vi "Main.vi"() -> ()   [LabVIEW 2019, in "MainController.lvlib"]
doc: "This Continuous Measurement sample project is based on the Queued Message Handler template.\n\nThe Event Handling Loop generates messages based on user interface actions.\n\nThe Message Handling Loop processes messages generated by the Event Handling Loop, or by other messages. There are also Acquisition and Logging message handling loop subVIs, and a chart updating loop."
uses:
  MainController/MainController.lvlib
  MainController/Cluster - MainData.ctl
  MainController/All Message Queues.ctl
  MainController/Cluster - MainControllerMessage.ctl
  MainController/Enum - MainState.ctl
  AutoMode/Cluster - AutoModeMessage.ctl
  AutoMode/Enum - AutoModeState.ctl
  ManualMode/Cluster - ManualModeMessageCluster.ctl
  ManualMode/Enum - ManualModeMessage.ctl
  Settings/CTL_MessageCluster.ctl
  Settings/CTL_SettingsMessage.ctl
  MainController/Cluster - HardwareConfiguration.ctl
  MainController/Cluster - LoggingConfiguration.ctl
  MainController/Cluster - TestSettings.ctl
  MainController/UI State.ctl
  MainController/UI Data.ctl
  Settings/Cluster - Settings.ctl
  <vilib>/Utility/error.llb/DialogType.ctl
  <vilib>/Utility/error.llb/Error Cluster From Error Code.vi
  <vilib>/ErrorRing/Error Ring.xnode
  Settings/Settings.lvlib
  support/User Event - Stop/User Event - Stop.lvlib
  ManualMode/ManualMode.lvlib
  AutoMode/AutoMode.lvlib
  support/User Interface/UserInterface.lvlib
  Dialogs/Flyout/Flyout.lvlib
panel:
  in  "ManualMode":bool
  in  "Test Report":bool
  in  "AutoMode":bool
  in  "HiliteNav":bool
  out "NavPaneTitle":string
  in  "Back":bool
  in  "Exit":bool
  in  "Global Navigation":bool
  in  "Settings":bool
  in  "COM":refnum<visa-resource-name>
  out "Mark 10":bool
  in  "Connect":bool
  in  "Titlebar":bool
  in  "Maximize":bool
  in  "Minimize":bool
  in  "Close":bool
  in  "CommandBar":T1
  out "Auto Mode":bool
  # "Auto Mode"
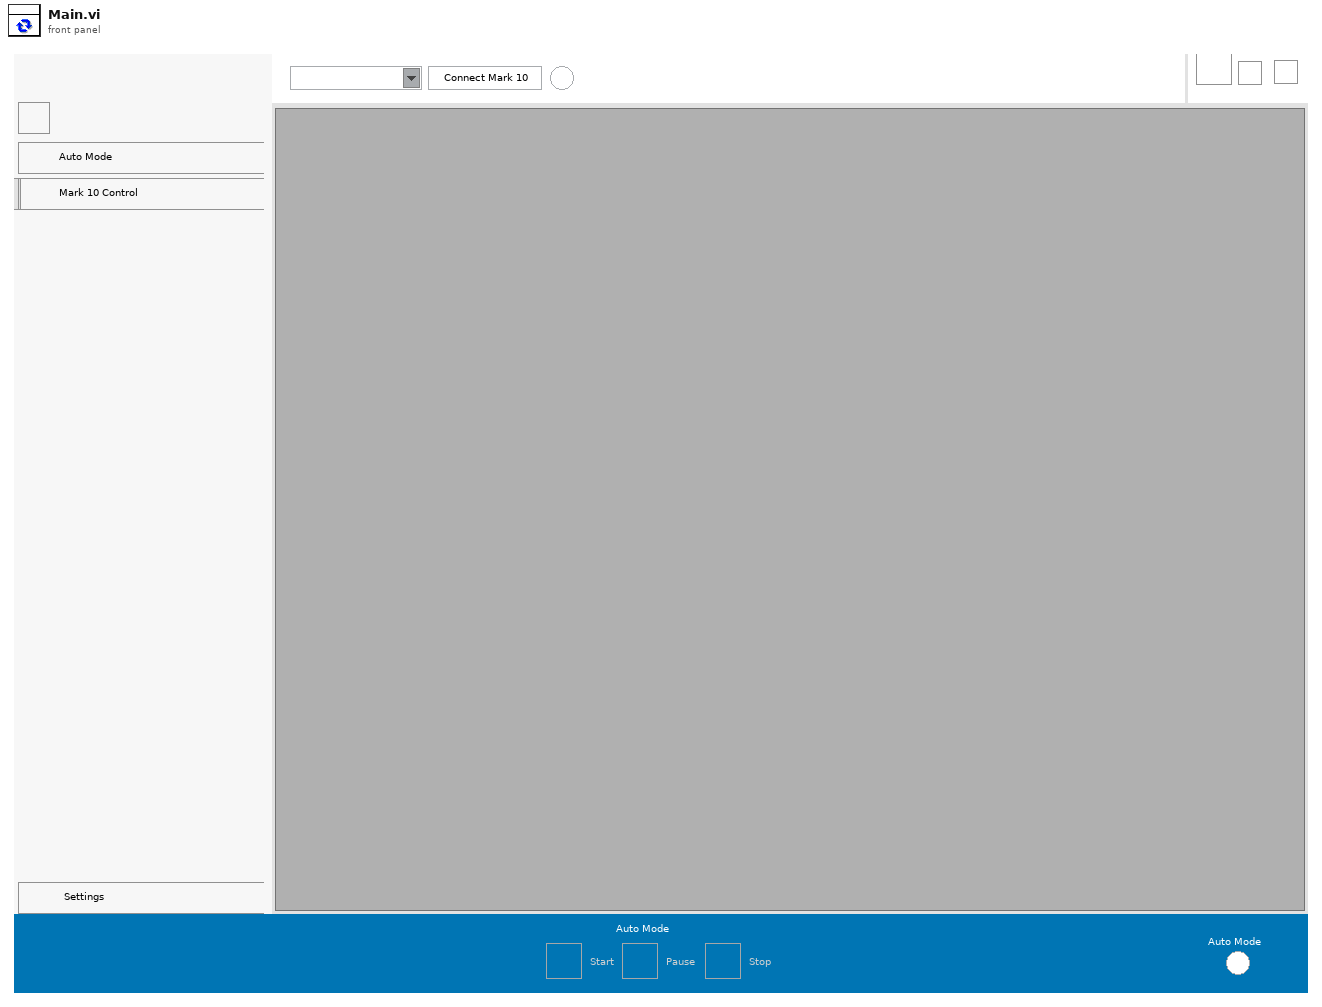
[diagram p1: front panel]
types:
  T1 = cluster{"StartCycleTest":bool, "PauseCycleTest":bool, "StopCycleTest":bool}
  T2 = typedef "MainController.lvlib/Cluster - MainData.ctl" = cluster{"MessageQueues":T3, "HardwareConfig":T4, "LoggingConfig":T5, "TestSettings":T6, "UI State":T7, "UIRefs":T8}
  T3 = typedef "MainController.lvlib/All Message Queues.ctl" = cluster{"Main":refnum<queue>, "AutoMode":refnum<queue>, "ManualMode":refnum<queue>, "Settings":refnum<queue>}
  T4 = typedef "MainController.lvlib/Cluster - HardwareConfiguration.ctl" = cluster{"Mark10COM":refnum<visa-resource-name>, "IsConnected":bool}
  T5 = typedef "MainController.lvlib/Cluster - LoggingConfiguration.ctl" = cluster{"Log File Base Path":path, "Comments ":string, "Operator":string, "File Name":string, "Description":string}
  T6 = typedef "MainController.lvlib/Cluster - TestSettings.ctl" = cluster{"Sample":u32, "Applicator Prefix":string, "Winding Distance":dbl, "Winding Speed":dbl, "Dwell Time":dbl, "Auto Increment Sample":bool, "Output Data Path":path, "File Base Path":path, "Manual Return To Zero":bool}
  T7 = typedef "MainController.lvlib/UI State.ctl" = enum16{"Idle", "AutoIdle", "AutoRunning", "ManualMode", "Settings"}
  T8 = typedef "MainController.lvlib/UI Data.ctl" = cluster{"Start Ref":refnum<vi>, "Stop Ref":refnum<vi>, "Settings Ref":refnum<vi>, "Subpanel":refnum<vi>, "HiliteNav Ref":refnum<vi>, "PauseCycle":refnum<vi>, "Connect":refnum<vi>, "ConnectionFbk":refnum<vi>, "AutoMode":refnum<vi>, "ManualMode":refnum<vi>}
  T9 = typedef "MainController.lvlib/Enum - MainState.ctl" = enum16{"Initialize", "InitUIRefs", "LaunchSettings", "LaunchAutoMode", "LaunchManualMode", "LaunchTestReport", "ConnectHardware", "DisconnectHardware", "HiliteNavItems", "StartAutoMode", "PauseAutoMode", "StopAutoMode", "ShowFlyout", "HideFlyout", "BroadcastSettings", "PickupTestSettings", "BroadcastHW", "AutoTestDone", "DAQStatus", "UpdateCommandBar", "Error", "RecieveError", "Exit"}
  T10 = enum32{"Invalid", "Standard", "Closed", "Hidden", "Minimized", "Maximized"}
  T11 = typedef "AutoMode.lvlib/Enum - AutoModeState.ctl" = enum16{"Initialize", "Idle", "UpdateConfig", "UpdateHWConfig", "BroadcastSettings", "Start", "CheckValidReportPath", "Winding", "WaitForWinding", "Unwind", "WaitForUnwind", "Stop", "Abort", "WriteDataToFile", "EventTriggered", "GenerateFilePath", "ZeroPosition", "GotoZero", "Error", "Exit"}
  T12 = typedef "Settings.lvlib/Cluster - Settings.ctl" = cluster{"Hardware Configuration":T4, "TestSettings":T6}
  T13 = typedef "ManualMode.lvlib/Enum - ManualModeMessage.ctl" = enum16{"Initialize", "Idle", "Start", "Stop", "Pause", "Resume", "BroadcastPreCollection", "MoveCCW", "MoveCW", "StopMove", "SetZero", "GotoZero", "UpdateHW", "SendMark10Cmd", "ReadPosition", "ReadTorque", "ReadStatus", "Error", "Exit"}
  T14 = typedef "Settings.lvlib/CTL_SettingsMessage.ctl" = enum16{"Inititalize", "Idle", "LoadSettings", "SaveSettings", "Exit"}
  T15 = typedef "DialogType.ctl" = u16
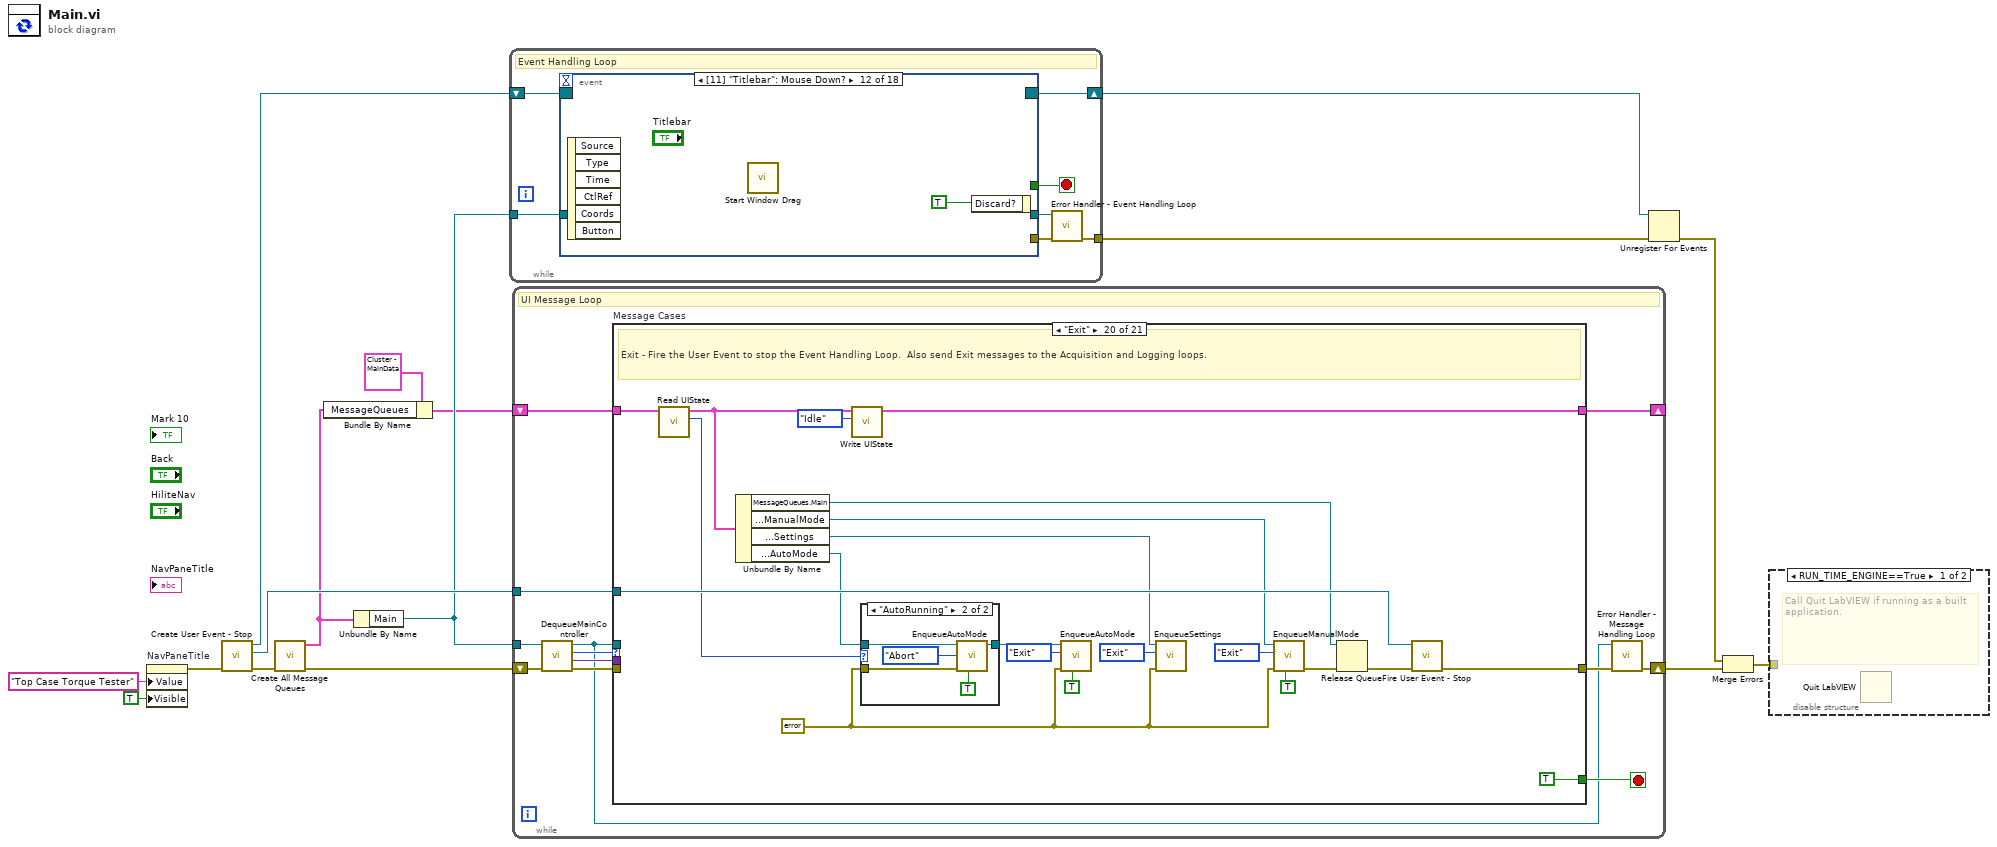
[diagram p0: block diagram]
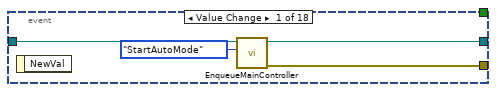
[diagram p3: hidden frame]
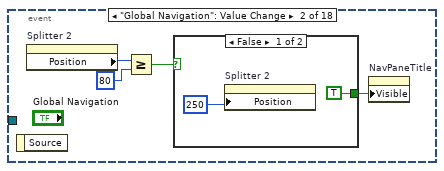
[diagram p4: hidden frame]
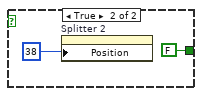
[diagram p5: hidden frame]
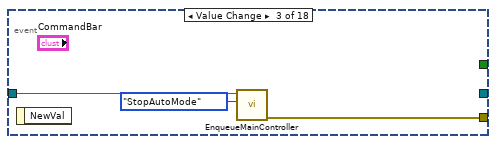
[diagram p6: hidden frame]
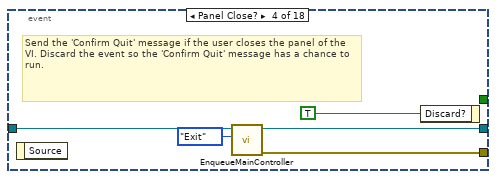
[diagram p7: hidden frame]
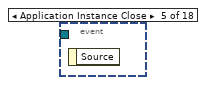
[diagram p8: hidden frame]
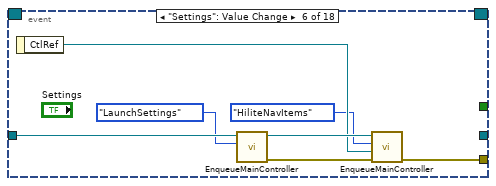
[diagram p9: hidden frame]
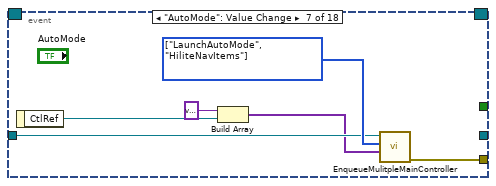
[diagram p10: hidden frame]
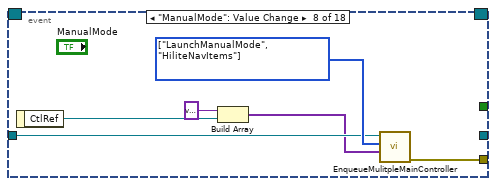
[diagram p11: hidden frame]
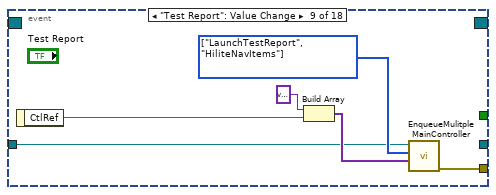
[diagram p12: hidden frame]
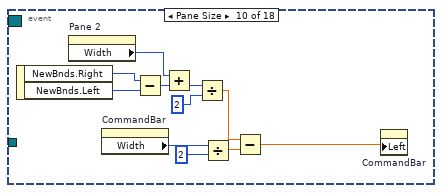
[diagram p13: hidden frame]
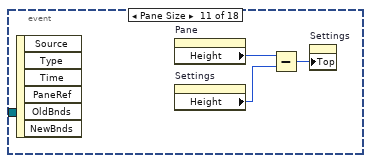
[diagram p14: hidden frame]
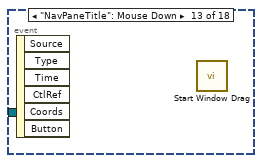
[diagram p15: hidden frame]
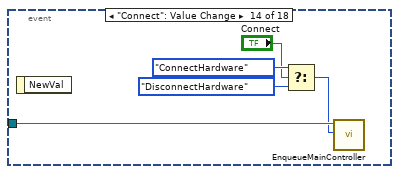
[diagram p16: hidden frame]
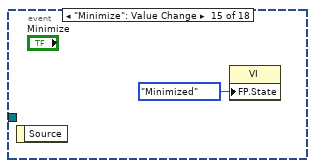
[diagram p17: hidden frame]
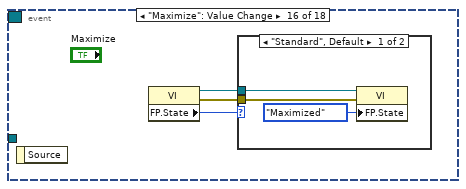
[diagram p18: hidden frame]
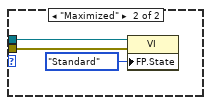
[diagram p19: hidden frame]
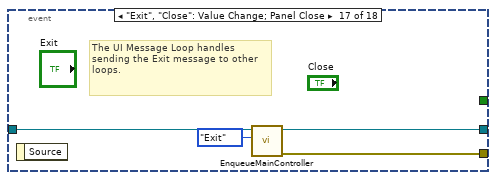
[diagram p20: hidden frame]
diagram:
  n1 = property on="NavPaneTitle" class="Str"("Value"="Top Case Torque Tester" ("NavPaneTitle"), "Visible"=TRUE) -> (error out=w5:errorcluster)  [unwired: 2 in, 1 out]
  n2 = call "Create User Event - Stop.vi"("error in (no error)"=w5) -> ("error out"=w12:errorcluster, "User Event - Stop"=w13:refnum<user-event>, "Stop Event Registration Refnum"=w14:refnum<event-registration>)  [unwired: 8 in]
  n3 = call "Create All Message Queues.vi"("error in (no error)"=w12) -> ("error out"=w7:errorcluster, "Message Queues out"=w3:T3)  [unwired: 9 in]
  n4 = Bundle By Name(cluster=T2 {"MessageQueues"={"Main"=refnum, "AutoMode"=refnum, "ManualMode"=refnum, "Settings"=refnum}, "HardwareConfig"={"Mark10COM"="", "IsConnected"=FALSE}, "LoggingConfig"={"Log File Base Path"=path "", "Comments "="", "Operator"="", "File Name"="", "Description"=""}, "TestSettings"={"Sample"=0, "Applicator Prefix"="", "Winding Distance"=0.0, "Winding Speed"=0.0, "Dwell Time"=0.0, "Auto Increment Sample"=FALSE, "Output Data Path"=path "", "File Base Path"=path "", "Manual Return To Zero"=FALSE}, "UI State"=enum."Idle", "UIRefs"={"Start Ref"=refnum, "Stop Ref"=refnum, "Settings Ref"=refnum, "Subpanel"=refnum, "HiliteNav Ref"=refnum, "PauseCycle"=refnum, "Connect"=refnum, "ConnectionFbk"=refnum, "AutoMode"=refnum, "ManualMode"=refnum}} ("MainData"), "MessageQueues"=w3) -> (w2:T2)
  n5 = Unbundle By Name(w3) -> ("Main"=w6:refnum<queue>)
  n6 = while {
    tunnel: w6 -> [w22]
    tunnel: [w18] -> w15
    shift-right: [w21] -> w10
    shift-left: w14 -> [w23]
    stop <- w20 stop-if-true
    # "Event Handling Loop"
    n7 = event shown="[11] \"Titlebar\": Mouse Down?" {
      selector: w23 -> [_ _ _ _ _ _ _ _ _ _ _ _ _ _ _ _ _ _]
      dyn-events: [_ _ _ _ _ _ _ _ _ _ _ _ _ _ _ _ _ _] -> w21
      timeout: _ -> [_ _ _ _ _ _ _ _ _ _ _ _ _ _ _ _ _ _]
      tunnel: [_ _ _ _ _ _ _ _ _ _ _ _ _ _ _ _ _ TRUE ("Discard?")] -> w20
      tunnel: w22 -> [w25 _ w37 w42 _ w50 w54 w60 w63 _ _ _ _ w88 _ _ w101 _]
      tunnel: [w27 _ w38 w41 _ w47 w56 w62 w68 _ _ _ _ _ _ _ w102 _] -> w19
      tunnel: [w26 _ _ w40 _ _ _ _ _ _ _ _ _ _ _ _ w99 _] -> w17
      event "CommandBar.StartCycleTest": Value Change {
        n8 = event-data() -> ()  [unwired: 1 in, 1 out]
        n9 = call "EnqueueMainController.vi"("Message"=Enum_-_MainState."StartAutoMode", "MainQueue"=w25) -> ("error out"=w27:errorcluster, "MainQueue out"=w26:refnum<queue>)  [unwired: 7 in, 1 out]
      }
      event "Global Navigation": Value Change {
        n10 = event-data() -> ()  [unwired: 1 in, 1 out]
        n11 = property on="Splitter 2" class="Splitter"() -> ("Position"=w29:i32)  [unwired: 2 in, 2 out]
        n12 = Greater Or Equal?(x=w29, y=80) -> (x >= y?=w30:bool)
        n13 = case shown="False" w30 {
          tunnel: [TRUE FALSE] -> w28
          frame False {
            n14 = property on="Splitter 2" class="Splitter"("Position"=250 ("Splitter Position")) -> ()  [unwired: 2 in, 2 out]
          }
          frame True {
            n15 = property on="Splitter 2" class="Splitter"("Position"=38 ("Splitter Position")) -> ()  [unwired: 2 in, 2 out]
          }
        }
        n16 = property on="NavPaneTitle" class="Str"("Visible"=w28) -> ()  [unwired: 2 in, 2 out]
      }
      event "CommandBar.StopCycleTest": Value Change {
        n17 = event-data() -> ()  [unwired: 1 in, 1 out]
        n18 = call "EnqueueMainController.vi"("Message"=Enum_-_MainState."StopAutoMode", "MainQueue"=w37) -> ("error out"=w38:errorcluster)  [unwired: 7 in, 2 out]
      }
      event Panel Close? {
        # "Send the 'Confirm Quit' message if the user closes the panel of the VI. Discard the event so the 'Confirm Quit' message has a chance to run."
        n19 = event-data() -> ()  [unwired: 1 in, 1 out]
        n20 = call "EnqueueMainController.vi"("Message"=Enum_-_MainState."Exit", "MainQueue"=w42) -> ("error out"=w41:errorcluster, "MainQueue out"=w40:refnum<queue>)  [unwired: 7 in, 1 out]
        n21 = event-data("Discard?"=TRUE) -> ()  [unwired: 1 in, 1 out]
      }
      event Application Instance Close {
        n22 = event-data() -> ()  [unwired: 1 in, 1 out]
      }
      event "Settings": Value Change {
        n23 = event-data() -> ("CtlRef"=w46:refnum<vi>)  [unwired: 1 in]
        n24 = call "EnqueueMainController.vi"("Message"=Enum_-_MainState."LaunchSettings", "MainQueue"=w50) -> ("error out"=w48:errorcluster, "MainQueue out"=w49:refnum<queue>)  [unwired: 7 in, 1 out]
        n25 = call "EnqueueMainController.vi"("error in (no error)"=w48, "Data"=w46, "Message"=Enum_-_MainState."HiliteNavItems", "MainQueue"=w49) -> ("error out"=w47:errorcluster)  [unwired: 5 in, 2 out]
      }
      event "AutoMode": Value Change {
        w55 = T9[] [enum."LaunchAutoMode", enum."HiliteNavItems"] items=["Initialize", "InitUIRefs", "LaunchSettings", "LaunchAutoMode", "LaunchManualMode", "LaunchTestReport", "ConnectHardware", "DisconnectHardware", "HiliteNavItems", "StartAutoMode", "PauseAutoMode", "StopAutoMode", "ShowFlyout", "HideFlyout", "BroadcastSettings", "PickupTestSettings", "BroadcastHW", "AutoTestDone", "DAQStatus", "UpdateCommandBar", "Error", "RecieveError", "Exit"] ("Messages")
        n26 = event-data() -> ("CtlRef"=w53:refnum<vi>)  [unwired: 1 in]
        n27 = Build Array(variant, w53) -> (w52:variant[])
        n28 = call "EnqueueMulitpleMainController.vi"("Data"=w52, "Messages"=w55, "MainQueue"=w54) -> ("error out"=w56:errorcluster)  [unwired: 6 in, 2 out]
      }
      event "ManualMode": Value Change {
        w61 = T9[] [enum."LaunchManualMode", enum."HiliteNavItems"] items=["Initialize", "InitUIRefs", "LaunchSettings", "LaunchAutoMode", "LaunchManualMode", "LaunchTestReport", "ConnectHardware", "DisconnectHardware", "HiliteNavItems", "StartAutoMode", "PauseAutoMode", "StopAutoMode", "ShowFlyout", "HideFlyout", "BroadcastSettings", "PickupTestSettings", "BroadcastHW", "AutoTestDone", "DAQStatus", "UpdateCommandBar", "Error", "RecieveError", "Exit"] ("Messages")
        n29 = event-data() -> ("CtlRef"=w59:refnum<vi>)  [unwired: 1 in]
        n30 = Build Array(variant, w59) -> (w58:variant[])
        n31 = call "EnqueueMulitpleMainController.vi"("Data"=w58, "Messages"=w61, "MainQueue"=w60) -> ("error out"=w62:errorcluster)  [unwired: 6 in, 2 out]
      }
      event "Test Report": Value Change {
        w67 = T9[] [enum."LaunchTestReport", enum."HiliteNavItems"] items=["Initialize", "InitUIRefs", "LaunchSettings", "LaunchAutoMode", "LaunchManualMode", "LaunchTestReport", "ConnectHardware", "DisconnectHardware", "HiliteNavItems", "StartAutoMode", "PauseAutoMode", "StopAutoMode", "ShowFlyout", "HideFlyout", "BroadcastSettings", "PickupTestSettings", "BroadcastHW", "AutoTestDone", "DAQStatus", "UpdateCommandBar", "Error", "RecieveError", "Exit"] ("Messages")
        n32 = event-data() -> ("CtlRef"=w66:refnum<vi>)  [unwired: 1 in]
        n33 = Build Array(variant, w66) -> (w65:variant[])
        n34 = call "EnqueueMulitpleMainController.vi"("Data"=w65, "Messages"=w67, "MainQueue"=w63) -> ("error out"=w68:errorcluster)  [unwired: 6 in, 2 out]
      }
      event Pane Size {
        n35 = event-data() -> ("NewBnds.Right"=w78:i16, "NewBnds.Left"=w79:i16)  [unwired: 1 in]
        n36 = property on="Pane 2" class="Pane"() -> ("Width"=w69:u32)  [unwired: 2 in, 2 out]
        n37 = property on="CommandBar" class="Clust (strict)"() -> ("Width"=w75:u32)  [unwired: 2 in, 2 out]
        n38 = Subtract(x=w78, y=w79) -> (x-y=w77:i16)
        n39 = Add(x=w69, y=w77) -> (x+y=w70:u32)
        n40 = Divide(x=w70, y=i16 2) -> (x/y=w73:dbl)
        n41 = Divide(x=w75, y=u32 2) -> (x/y=w72:dbl)
        n42 = Subtract(x=w73, y=w72) -> (x-y=w71:dbl)
        n43 = property on="CommandBar" class="Clust (strict)"("Left"=w71) -> ()  [unwired: 2 in, 2 out]
      }
      event Pane Size {
        n44 = event-data() -> ()  [unwired: 1 in, 6 out]
        n45 = property on="Pane" class="Pane"() -> ("Height"=w80:u32)  [unwired: 2 in, 2 out]
        n46 = property on="Settings" class="Bool"() -> ("Height"=w82:u32)  [unwired: 2 in, 2 out]
        n47 = Subtract(x=w80, y=w82) -> (x-y=w81:u32)
        n48 = property on="Settings" class="Bool"("Top"=w81) -> ()  [unwired: 2 in, 2 out]
      }
      event "Titlebar": Mouse Down? {
        n49 = event-data() -> ()  [unwired: 1 in, 6 out]
        n50 = call "Start Window Drag.vi"() -> ()  [unwired: 10 in, 2 out]
        n51 = event-data("Discard?"=TRUE) -> ()  [unwired: 1 in, 1 out]
      }
      event "NavPaneTitle": Mouse Down {
        n52 = event-data() -> ()  [unwired: 1 in, 6 out]
        n53 = call "Start Window Drag.vi"() -> ()  [unwired: 10 in, 2 out]
      }
      event "Connect": Value Change {
        n54 = event-data() -> ()  [unwired: 1 in, 1 out]
        n55 = Select(t=Enum_-_MainState."ConnectHardware" ("Message"), s="Connect", f=Enum_-_MainState."DisconnectHardware" ("Message")) -> (s? t:f=w84:T9)
        n56 = call "EnqueueMainController.vi"("Message"=w84, "MainQueue"=w88) -> ()  [unwired: 7 in, 3 out]
      }
      event "Minimize": Value Change {
        n57 = event-data() -> ()  [unwired: 1 in, 1 out]
        n58 = property class="VI"("FP.State"=T10."Minimized" ("Front Panel Window:State")) -> ()  [unwired: 2 in, 2 out]
      }
      event "Maximize": Value Change {
        n59 = event-data() -> ()  [unwired: 1 in, 1 out]
        n60 = property class="VI"() -> (reference out=w91:refnum<vi>, error out=w92:errorcluster, "FP.State"=w90:T10)  [unwired: 2 in]
        n61 = case shown="\"Standard\", Default" w90 {
          tunnel: w92 -> [w94 w97]
          tunnel: w91 -> [w93 w96]
          frame "Standard", Default {
            n62 = property class="VI"(reference=w93, error in=w94, "FP.State"=T10."Maximized" ("Front Panel Window:State")) -> ()  [unwired: 2 out]
          }
          frame "Maximized" {
            n63 = property class="VI"(reference=w96, error in=w97, "FP.State"=T10."Standard" ("Front Panel Window:State")) -> ()  [unwired: 2 out]
          }
        }
      }
      event "Exit", "Close": Value Change; Panel Close {
        # "The UI Message Loop handles sending the Exit message to other loops."
        n64 = event-data() -> ()  [unwired: 1 in, 1 out]
        n65 = call "EnqueueMainController.vi"("Message"=Enum_-_MainState."Exit", "MainQueue"=w101) -> ("error out"=w102:errorcluster, "MainQueue out"=w99:refnum<queue>)  [unwired: 7 in, 1 out]
      }
      event User Event {
        # "The Message Handling Loop processed an \"Exit\" message, which fired this event to stop the Event Handling Loop."
        n66 = event-data() -> ()  [unwired: 1 in, 1 out]
      }
    }
    n67 = call "Error Handler - Event Handling Loop.vi"("error in (no error)"=w19, "Message Queue"=w17) -> ("dup error in"=w18:errorcluster)  [unwired: 8 in, 1 out]
  }
  n68 = while {
    tunnel: w6 -> [w110]
    tunnel: w13 -> [w114]
    shift-right: [w107] -> w16
    shift-left: w7 -> [w113]
    shift-right: [w105] -> _
    shift-left: w2 -> [w109]
    stop <- w115 stop-if-true
    # "UI Message Loop"
    n69 = call "DequeueMainController.vi"("error in (no error)"=w113, "MainQueue"=w110) -> ("error out"=w112:errorcluster, "Data"=w111:variant, "Message"=w106:T9, "MainQueue out"=w104:refnum<queue>)  [unwired: 5 in, 1 out]
    n70 = case "Message Cases" shown="\"Exit\"" w106 {
      selector: w106 -> [_ _ _ _ _ _ _ _ _ _ _ _ _ _ _ _ _ _ _ _ w342]
      tunnel: w104 -> [_ _ _ _ _ _ _ _ _ _ _ _ _ _ _ _ w268 _ _ _ _]
      tunnel: w112 -> [w119 _ w149 w156 w161 w165 w169 w176 w181 w192 w197 w207 w212 w224 w232 _ w271 w280 w287 _ _]
      tunnel: [w118 _ w146 w155 w160 w162 w168 w175 w177 w193 w196 w201 w211 w218 w231 _ w269 w277 w284 w332 w343] -> w108
      tunnel: [_ _ _ _ _ _ _ _ _ _ _ _ _ _ _ _ _ _ _ TRUE _] -> w115
      tunnel: w111 -> [_ _ _ _ _ _ _ _ _ w189 _ w205 w210 w222 _ _ _ w279 w286 _ _]
      tunnel: w114 -> [_ _ _ _ _ _ _ _ _ _ _ _ _ _ _ _ _ _ _ w333 _]
      tunnel: [w116 w124 w147 w153 w158 w164 w166 w174 w179 w183 w194 w198 w208 w216 w226 w242 w266 w276 w281 w325 w341] -> w105
      tunnel: w109 -> [w117 w126 w148 w154 w159 w163 w167 w170 w180 w183 w194 w198 w208 w220 w230 w243 w270 w276 w281 w326 w341]
      frame "Initialize" {
        # "Initialize - Get configuration settings, then message the UI to initialize, and broadcast the settings to the other message loops."
        n71 = call "Initialize.vi"("Error In"=w119, "MainData"=w117) -> ("Error Out"=w118:errorcluster, "MainData out"=w116:T2)  [unwired: 8 in]
        n72 = property on="Pane" class="Pane"() -> ("Height"=w122:u32)  [unwired: 2 in, 2 out]
        n73 = property on="Settings" class="Bool"() -> ("Height"=w120:u32)  [unwired: 2 in, 2 out]
        n74 = Subtract(x=w122, y=w120) -> (x-y=w121:u32)
        n75 = property on="Settings" class="Bool"("Top"=w121) -> ()  [unwired: 2 in, 2 out]
      }
      frame "InitUIRefs" {
        # "Init UI Refs - Store control references for UI controls.  Also enable/disable controls appropriately."
        n76 = control-ref of="StartCycleTest"() -> (w132:refnum<vi>)
        n77 = control-ref of="PauseCycleTest"() -> (w135:refnum<vi>)
        n78 = control-ref of="StopCycleTest"() -> (w136:refnum<vi>)
        n79 = control-ref of="Settings"() -> (w140:refnum<vi>)
        n80 = control-ref of="Connect"() -> (w130:refnum<vi>)
        n81 = control-ref of="ConnectionFbk"() -> (w129:refnum<vi>)
        n82 = Build Array(w140) -> (w142:refnum<vi>[])
        n83 = call "Set Enable State on Multiple Controls.vi"("Enable?"=TRUE, "Controls"=w142) -> ()  [unwired: 10 in]
        n84 = Build Array(w132, w135, w136) -> (w139:refnum<vi>[])
        n85 = call "Set Enable State on Multiple Controls.vi"("Enable?"=FALSE, "Controls"=w139) -> ()  [unwired: 10 in]
        n86 = control-ref of="Sub Panel"() -> (w137:refnum<vi>)
        n87 = control-ref of="HiliteNav"() -> (w138:refnum<vi>)
        n88 = control-ref of="AutoMode"() -> (w128:refnum<vi>)
        n89 = control-ref of="ManualMode"() -> (w131:refnum<vi>)
        n90 = property class="VI"("Front Panel.Closeable"=TRUE ("Front Panel Window:Closeable")) -> ()  [unwired: 2 in, 2 out]
        n91 = Bundle By Name(cluster=w126, "UIRefs.Start Ref"=w132, "UIRefs.PauseCycle"=w135, "UIRefs.Stop Ref"=w136, "UIRefs.Settings Ref"=w140, "UIRefs.Subpanel"=w137, "UIRefs.HiliteNav Ref"=w138, "UIRefs.AutoMode"=w128, "UIRefs.ManualMode"=w131, "UIRefs.Connect"=w130, "UIRefs.ConnectionFbk"=w129) -> (w125:T2)
        n92 = property on="Flyout" class="SubPnl"("Visible"=FALSE) -> ()  [unwired: 2 in, 2 out]
        n93 = local write "Mark 10"(FALSE ("DAQ")) -> ()
        n94 = property on="Connect" class="Bool (strict)"("Value"=FALSE ("Connect")) -> ()  [unwired: 2 in, 2 out]
        n95 = call "Write UIState.vi"("UI State"=UI_State."Idle", "MainData"=w125) -> ("MainData out"=w124:T2)  [unwired: 9 in]
      }
      frame "StartAutoMode" {
        n96 = call "StartAutoMode.vi"("error in (no error)"=w149, "MainData"=w148) -> ("error out"=w145:errorcluster, "MainData out"=w147:T2)  [unwired: 8 in]
        n97 = flat-sequence {
          tunnel: [w150] -> w146
          tunnel: w145 -> [w150]
          frame #0 {
            n98 = property on="StartCycleTest" class="Bool (strict)"("Value"=FALSE) -> ()  [unwired: 2 in, 2 out]
            "Auto Mode" <- TRUE ("Cycle Test")
          }
        }
      }
      frame "StopAutoMode" {
        w157 = FALSE ("Value")
        # "Stop - Enable/Disable buttons appropriately for an acquisition that has stopped, and update status display."
        n99 = property on="StopCycleTest" class="Bool (strict)"("Value"=w157) -> ()  [unwired: 2 in, 2 out]
        n100 = property on="Auto Mode" class="Bool (strict)"("Value"=w157) -> ()  [unwired: 2 in, 2 out]
        n101 = call "StopAutoMode.vi"("error in (no error)"=w156, "MainData"=w154) -> ("error out"=w155:errorcluster, "MainData out"=w153:T2)  [unwired: 8 in]
      }
      frame "LaunchAutoMode" {
        n102 = call "LaunchAutoMode.vi"("error in (no error)"=w161, "MainData"=w159) -> ("error out"=w160:errorcluster, "MainData out"=w158:T2)  [unwired: 8 in]
      }
      frame "LaunchSettings" {
        # "Launch the Settings Dialog when the user clicks the 'Settings' button."
        n103 = call "LaunchSettingsPanel.vi"("error in (no error)"=w165, "MainData"=w163) -> ("error out"=w162:errorcluster, "MainData out"=w164:T2)  [unwired: 8 in]
      }
      frame "LaunchManualMode" {
        n104 = call "LaunchManualMode.vi"("error in (no error)"=w169, "MainData"=w167) -> ("error out"=w168:errorcluster, "MainData out"=w166:T2)  [unwired: 8 in]
      }
      frame "ConnectHardware" {
        n105 = Bundle By Name(cluster=w170, "HardwareConfig.Mark10COM"="COM") -> (w171:T2)
        n106 = call "ConnectHardware.vi"("Error In"=w176, "MainData"=w171) -> ("Error Out"=w175:errorcluster, "MainData out"=w174:T2)  [unwired: 8 in]
        n107 = Unbundle By Name(w174) -> ("HardwareConfig.IsConnected"=w173:bool)
        n108 = property on="Mark 10" class="Bool (strict)"(error in=w175, "Value"=w173) -> ()  [unwired: 1 in, 2 out]
        n109 = property on="Connect" class="Bool (strict)"(error in=w175, "Value"=w173) -> ()  [unwired: 1 in, 2 out]
      }
      frame "DisconnectHardware" {
        n110 = call "DisconnectHardware.vi"("Error In"=w181, "MainData"=w180) -> ("Error Out"=w178:errorcluster, "MainData out"=w179:T2)  [unwired: 8 in]
        n111 = property on="Mark 10" class="Bool (strict)"(error in=w178, "Value"=FALSE ("Mark 10")) -> (error out=w177:errorcluster)  [unwired: 1 in, 1 out]
      }
      frame "ShowFlyout" {
        n112 = Unbundle By Name(w183) -> ("MessageQueues.Main"=w184:refnum<queue>)
        n113 = Variant To Data(error in=w192, type=cluster{"Message":string, "Timeout":dbl} {"Message"="", "Timeout"=0.0}, Variant=w189) -> (data=w187:cluster{"Message":string, "Timeout":dbl}, error out=w190:errorcluster)
        n114 = Unbundle By Name(w187) -> ("Message"=w185:string, "Timeout"=w186:dbl)
        n115 = control-ref of="Flyout"() -> (w191:refnum<vi>)
        n116 = call "ShowFlyout.vi"("MainUI"=w184, "error in (no error)"=w190, "Subpanel"=w191, "Timeout"=w186, "Message"=w185) -> ("error out"=w193:errorcluster)  [unwired: 6 in]
      }
      frame "HideFlyout" {
        n117 = control-ref of="Flyout"() -> (w195:refnum<vi>)
        n118 = invoke class="SubPnl" method="Remove VI"(reference=w195, error in=w197) -> (error out=w196:errorcluster)  [unwired: 1 in, 2 out]
      }
      frame "HiliteNavItems" {
        n119 = Variant To Data(error in=w207, type=refnum<vi> refnum ("CtlRef"), Variant=w205) -> (data=w202:refnum<vi>, error out=w206:errorcluster)
        n120 = property class="Bool"(reference=w202, error in=w206) -> (error out=w203:errorcluster, "Top"=w199:i32)  [unwired: 1 out]
        n121 = Unbundle By Name(w198) -> ("UIRefs.HiliteNav Ref"=w200:refnum<vi>)
        n122 = property class="Bool"(reference=w200, error in=w203, "Top"=w199) -> (error out=w201:errorcluster)  [unwired: 1 out]
      }
      frame "DAQStatus" {
        n123 = Variant To Data(error in=w212, type=FALSE, Variant=w210) -> (error out=w211:errorcluster)  [unwired: 1 out]
      }
      frame "BroadcastSettings" {
        n124 = Variant To Data(error in=w224, type=T12 {"Hardware Configuration"={"Mark10COM"="", "IsConnected"=FALSE}, "TestSettings"={"Sample"=0, "Applicator Prefix"="", "Winding Distance"=0.0, "Winding Speed"=0.0, "Dwell Time"=0.0, "Auto Increment Sample"=FALSE, "Output Data Path"=path "", "File Base Path"=path "", "Manual Return To Zero"=FALSE}} ("Settings in"), Variant=w222) -> (data=w217:T12, error out=w223:errorcluster)
        n125 = Unbundle By Name(w217) -> ("Hardware Configuration"=w219:T4, "TestSettings"=w213:T6)
        n126 = Bundle By Name(cluster=w220, "HardwareConfig"=w219, "TestSettings"=w213) -> (w216:T2)
        n127 = Unbundle By Name(w216) -> ("MessageQueues.AutoMode"=w215:refnum<queue>)
        n128 = call "EnqueueAutoMode.vi"("error in (no error)"=w223, "Data"=w213, "AutoState"=Enum_-_AutoModeState."UpdateConfig" ("CycleTestState"), "Queue in"=w215) -> ("error out"=w218:errorcluster)  [unwired: 6 in, 1 out]
      }
      frame "BroadcastHW" {
        n129 = call "Read UIState.vi"("MainData"=w230) -> ("UI State"=w225:T7, "MainData out"=w226:T2)  [unwired: 9 in]
        n130 = case shown="\"ManualMode\"" w225 {
          tunnel: [w234 w235] -> w233
          tunnel: w232 -> [w234 w240]
          tunnel: w230 -> [_ w239]
          frame Default {
          }
          frame "ManualMode" {
            n131 = Unbundle By Name(w239) -> ("MessageQueues.ManualMode"=w238:refnum<queue>, "HardwareConfig"=w236:T4)
            n132 = call "EnqueueManualMode.vi"("error in (no error)"=w240, "Data"=w236, "Message"=Enum_-_ManualModeMessage."Start", "queue"=w238) -> ("error out"=w235:errorcluster)  [unwired: 6 in, 1 out]
          }
        }
        n133 = Unbundle By Name(w226) -> ("MessageQueues.AutoMode"=w229:refnum<queue>, "HardwareConfig"=w228:T4)
        n134 = call "EnqueueAutoMode.vi"("error in (no error)"=w233, "Data"=w228, "AutoState"=Enum_-_AutoModeState."UpdateHWConfig", "Queue in"=w229) -> ("error out"=w231:errorcluster)  [unwired: 6 in, 1 out]
      }
      frame "UpdateCommandBar" {
        n135 = call "Read UIState.vi"("MainData"=w243) -> ("UI State"=w241:T7, "MainData out"=w242:T2)  [unwired: 9 in]
        n136 = case shown="\"AutoRunning\"" w241 {
          tunnel: w242 -> [w244 w251 w258]
          frame "AutoIdle" {
            n137 = Unbundle By Name(w244) -> ("HardwareConfig.IsConnected"=w248:bool)
            n138 = Unbundle By Name(w244) -> ("UIRefs.Start Ref"=w250:refnum<vi>, "UIRefs.Stop Ref"=w247:refnum<vi>)
            n139 = Build Array(w250) -> (w249:refnum<vi>[])
            n140 = Build Array(w247) -> (w246:refnum<vi>[])
            n141 = call "Set Enable State on Multiple Controls.vi"("Enable?"=w248, "Controls"=w249) -> ()  [unwired: 10 in]
            n142 = call "Set Enable State on Multiple Controls.vi"("Enable?"=FALSE, "Controls"=w246) -> ()  [unwired: 10 in]
          }
          frame "AutoRunning" {
            n143 = Unbundle By Name(w251) -> ("UIRefs.Start Ref"=w257:refnum<vi>, "UIRefs.Stop Ref"=w255:refnum<vi>)
            n144 = Build Array(w257) -> (w256:refnum<vi>[])
            n145 = Build Array(w255) -> (w254:refnum<vi>[])
            n146 = call "Set Enable State on Multiple Controls.vi"("Enable?"=FALSE, "Controls"=w256) -> ()  [unwired: 10 in]
            n147 = call "Set Enable State on Multiple Controls.vi"("Enable?"=TRUE, "Controls"=w254) -> ()  [unwired: 10 in]
          }
          frame "Idle", "ManualMode", "Settings", Default {
            n148 = Unbundle By Name(w258) -> ("UIRefs.Start Ref"=w264:refnum<vi>, "UIRefs.Stop Ref"=w262:refnum<vi>)
            n149 = Build Array(w264) -> (w263:refnum<vi>[])
            n150 = Build Array(w262) -> (w261:refnum<vi>[])
            n151 = call "Set Enable State on Multiple Controls.vi"("Enable?"=FALSE, "Controls"=w263) -> ()  [unwired: 10 in]
            n152 = call "Set Enable State on Multiple Controls.vi"("Enable?"=FALSE, "Controls"=w261) -> ()  [unwired: 10 in]
          }
        }
      }
      frame "AutoTestDone" {
        n153 = call "Write UIState.vi"("UI State"=UI_State."AutoIdle", "MainData"=w270) -> ("MainData out"=w266:T2)  [unwired: 9 in]
        n154 = call "EnqueueMainController.vi"("error in (no error)"=w271, "Message"=Enum_-_MainState."UpdateCommandBar", "MainQueue"=w268) -> ("error out"=w269:errorcluster)  [unwired: 6 in, 2 out]
      }
      frame "Error" {
        # "Error - Check the error message data and respond accordingly. This message is sent by the \"Error Handler\" VIs at the end of each loop in this application."
        n155 = Variant To Data(error in=w280, type=errorcluster {"status"=FALSE, "code"=0, "source"=""} ("error out"), Variant=w279) -> (data=w275:errorcluster, error out=w277:errorcluster)
        n156 = Unbundle By Name(w275) -> ("source"=w274:string)
        n157 = Concatenate Strings("Error!\n" ("string"), w274) -> (w273:string)
        n158 = call "MessageDialog.vi"("error in (no error)"=w275, "Message"=w273) -> ()  [unwired: 9 in, 1 out]
      }
      frame "RecieveError" {
        # "Recieve error from calling task."
        n159 = Variant To Data(error in=w287, type=errorcluster {"status"=FALSE, "code"=0, "source"=""} ("error out"), Variant=w286) -> (data=w282:errorcluster)  [unwired: 1 out]
        n160 = Unbundle By Name(w282) -> ("code"=w283:i32)
        n161 = case shown="Default" w283 {
          tunnel: w282 -> [_ _ w302]
          tunnel: [w291 w298 w305] -> w284
          tunnel: w281 -> [w293 w299 w304]
          frame -201003 {
            w289 = T9[] [enum."DisconnectHardware"] items=["Initialize", "InitUIRefs", "LaunchSettings", "LaunchAutoMode", "LaunchManualMode", "LaunchTestReport", "ConnectHardware", "DisconnectHardware", "HiliteNavItems", "StartAutoMode", "PauseAutoMode", "StopAutoMode", "ShowFlyout", "HideFlyout", "BroadcastSettings", "PickupTestSettings", "BroadcastHW", "AutoTestDone", "DAQStatus", "UpdateCommandBar", "Error", "RecieveError", "Exit"] ("Messages")
            # "DAQ Device cannot be accessed"
            n162 = Unbundle By Name(w293) -> ("MessageQueues.Main"=w292:refnum<queue>)
            n163 = call "EnqueueMulitpleMainController.vi"("error in (no error)"=errorcluster {"status"=FALSE, "code"=0, "source"=""}, "Messages"=w289, "MainQueue"=w292) -> ("error out"=w291:errorcluster)  [unwired: 6 in, 2 out]
            n164 = call "MessageDialog.vi"("Message"="Could not connect to DAQ.\nCheck power and USB connection." ("message")) -> ()  [unwired: 10 in, 1 out]
          }
          frame -200477 {
            w295 = T9[] [enum."DisconnectHardware"] items=["Initialize", "InitUIRefs", "LaunchSettings", "LaunchAutoMode", "LaunchManualMode", "LaunchTestReport", "ConnectHardware", "DisconnectHardware", "HiliteNavItems", "StartAutoMode", "PauseAutoMode", "StopAutoMode", "ShowFlyout", "HideFlyout", "BroadcastSettings", "PickupTestSettings", "BroadcastHW", "AutoTestDone", "DAQStatus", "UpdateCommandBar", "Error", "RecieveError", "Exit"] ("Messages")
            # "DAQ Configuration error"
            n165 = Unbundle By Name(w299) -> ("MessageQueues.Main"=w296:refnum<queue>)
            n166 = call "EnqueueMulitpleMainController.vi"("error in (no error)"=errorcluster {"status"=FALSE, "code"=0, "source"=""}, "Messages"=w295, "MainQueue"=w296) -> ("error out"=w298:errorcluster)  [unwired: 6 in, 2 out]
            n167 = call "MessageDialog.vi"("Message"="Unable to configure DAQ.\nCheck DAQ device name in Settings." ("message")) -> ()  [unwired: 10 in, 1 out]
          }
          frame Default {
            w303 = T15 4 items=["no dialog", "OK message", "continue or stop message", "OK message + warnings", "continue/stop + warnings"] ("type of dialog (OK msg:1)")
            n168 = call <vilib>:"Simple Error Handler.vi"("type of dialog (OK msg:1)"=w303, "error in (no error)"=w302) -> ("error?"=w300:bool, "error out"=w301:errorcluster)  [unwired: 3 in, 3 out]
            n169 = case shown="False" w300 {
              tunnel: [w311 errorcluster {"status"=FALSE, "code"=0, "source"=""} ("error IO")] -> w305
              tunnel: w304 -> [w310 _]
              tunnel: w301 -> [w308 _]
              frame False {
                n170 = Unbundle By Name(w310) -> ("MessageQueues.Main"=w309:refnum<queue>)
                n171 = call <vilib>:"Clear Errors.vi"("error in (no error)"=w308) -> ("error out"=w307:errorcluster)  [unwired: 5 in, 1 out]
                n172 = call "EnqueueMainController.vi"("Message"=Enum_-_MainState."Exit", "MainQueue"=w309) -> ("error out"=w312:errorcluster)  [unwired: 7 in, 2 out]
                n173 = Merge Errors(w312, w307) -> (w311:errorcluster)
              }
              frame True {
              }
            }
          }
        }
      }
      frame "Exit" {
        w319 = errorcluster {"status"=FALSE, "code"=0, "source"=""} ("error in (no error)")
        # "Exit - Fire the User Event to stop the Event Handling Loop.  Also send Exit messages to the Acquisition and Logging loops."
        n174 = call "Read UIState.vi"("MainData"=w326) -> ("UI State"=w320:T7, "MainData out"=w315:T2)  [unwired: 9 in]
        n175 = Unbundle By Name(w315) -> ("MessageQueues.Main"=w317:refnum<queue>, "MessageQueues.ManualMode"=w329:refnum<queue>, "MessageQueues.Settings"=w327:refnum<queue>, "MessageQueues.AutoMode"=w322:refnum<queue>)
        n176 = call "Write UIState.vi"("UI State"=UI_State."Idle", "MainData"=w315) -> ("MainData out"=w325:T2)  [unwired: 9 in]
        n177 = case shown="\"AutoRunning\"" w320 {
          tunnel: w319 -> [_ w340]
          tunnel: w322 -> [w335 w339]
          tunnel: [w335 w338] -> w321
          frame "Idle", Default {
          }
          frame "AutoRunning" {
            n178 = call "EnqueueAutoMode.vi"("Priority Message"=TRUE, "error in (no error)"=w340, "AutoState"=Enum_-_AutoModeState."Abort", "Queue in"=w339) -> ("queue out"=w338:refnum<queue>)  [unwired: 6 in, 1 out]
          }
        }
        n179 = call "EnqueueAutoMode.vi"("Priority Message"=TRUE, "error in (no error)"=w319, "AutoState"=Enum_-_AutoModeState."Exit" ("CycleTestState"), "Queue in"=w321) -> ()  [unwired: 6 in, 2 out]
        n180 = call "EnqueueSettings.vi"("error in (no error)"=w319, "Message"=CTL_SettingsMessage."Exit", "SettingsQueue"=w327) -> ()  [unwired: 7 in, 2 out]
        n181 = call "EnqueueManualMode.vi"("Priority?"=TRUE, "error in (no error)"=w319, "Message"=Enum_-_ManualModeMessage."Exit" ("PreCollectionMessage"), "queue"=w329) -> ("error out"=w318:errorcluster)  [unwired: 6 in, 1 out]
        n182 = Release Queue(queue=w317, error in (no error)=w318) -> (error out=w316:errorcluster)  [unwired: 1 in, 2 out]
        n183 = call "Fire User Event - Stop.vi"("error in (no error)"=w316, "User Event - Stop"=w333) -> ("error out"=w332:errorcluster)  [unwired: 9 in]
      }
      frame Default {
        # "'Default' case only runs if there is a message that isn't defined in any of the other cases.  Output a programming error."
        n184 = xnode "Error Ring"("parameter 0"=w342) -> ("error out"=w343:errorcluster)
      }
    }
    n185 = call "Error Handler - Message Handling Loop.vi"("error in (no error)"=w108, "Message Queue"=w104) -> ("dup error in"=w107:errorcluster)  [unwired: 8 in, 1 out]
  }
  n186 = Unregister For Events(event registration refnum=w10, error in=w15) -> (error out=w11:errorcluster)
  n187 = Merge Errors(w11, w16) -> (w1:errorcluster)
  n188 = disable-structure shown="RUN_TIME_ENGINE==True" {
    disable-tunnel: w1 -> [_ _]
    frame condition #0 {
      # "Call Quit LabVIEW if running as a built application."
      n189 = Quit LabVIEW() -> ()  [unwired: 1 in]
    }
    frame condition #1 (active) {
    }
  }
